vi "Doppler gating.vi"() -> ()   [LabVIEW 2022 SP3]
doc: "I. Description:\nThis example demonstrates how to use the timed loop to efficiently acquire a continuous amount of data (Waveform) using the DAQ devices internal clock and a counter to execute the timed loop only when all the data is available to Read.\n\nII. Instructions for Running:\n1. Select the physical channel to correspond to where your signal is input on the DAQ device. \n2. Enter the Source of Events. In this case we want the loop to execute on each AI sample clock pulse.\n3. Enter the counter you want to use to measure the events. In this example ctr0 is used as the default.\n4. Enter the minimum and maximum voltages.\nNote: For better accuracy try to match the input range to the expected voltage level of the measured signal.\n5. Select the number of samples to Read. Note: Because of the way this example uses the timed loop this parameter cannot be changed on-the-fly. \n6. Set the rate of the acquisition\nNote: The rate should be AT LEAST twice as fast as the maximum frequency component of the signal being acquired.\n\nIII. Block Diagram Steps:\n1. Create an Analog Input voltage channel.\n2. Set the timing type of the analog input task to Sample Clock. \n3. Call the DAQmx Create Timing Source (Digital Edge Counter) VI and specify the edge count to be the Samples to Read. What this does is cause the timed loop to only fire once it has received \"samples to read\" number of edges from the AI sample clock. This is an efficient use of CPU resources because the loop, and therefore the AI Read, will only execute once all of the samples are available.\n4. Call the Start VI to start the acquisition.\n5. Read the waveform once all the samples to read are available. In this approach the Read VI behaves in a \"non-blocking\" fashion, since it does not have to wait for samples to become available.\n6. Call the Clear Task VI to Clear the Task.\n7. Use the popup dialog box to display an error if any.\n\nIV. I/O Connections Overview:\nMake sure your signal input terminal matches the Physical Channel I/O Control. For further connection information, refer to your hardware reference manual."
uses:
  <vilib>/Utility/error.llb/DialogType.ctl
  <vilib>/Platform/TimedLoop/XDataNode/timing_clust.ctl
  <vilib>/Platform/TimedLoop/XDataNode/nitl_modes.ctl
  <vilib>/Platform/TimedLoop/XDataNode/wakeup.ctl
  <vilib>/DAQmx/read.llb/DAQmx Read.vi
  <vilib>/DAQmx/create/channels.llb/DAQmx Create Virtual Channel.vi
  <vilib>/DAQmx/configure/timing.llb/DAQmx Timing.vi
  <vilib>/DAQmx/create/timing.llb/DAQmx Create Timing Source.vi
  <vilib>/DAQmx/miscellaneous.llb/DAQmx Fill In Error Info.vi
  Instance          16 22Saved   Doppler gating .vi
  <vilib>/Platform/TimedLoop/XDataNode/XDataNode.xnode
  <vilib>/ptbypt/NI_PtbyPt.lvlib
  <vilib>/gmath/NI_Gmath.lvlib
  <vilib>/Platform/TimedLoop/XDataNode/XDNodeRunTimeDep.lvlib
panel:
  in  "window length":i32=500 caption="Samples to Read"
  in  "time increment":i32=100 caption="Samples to Read"
  out "Moving STFT":dbl[][](graph)
  in  "Counter":tag="Dev1/ctr0"
  in  "Source of Events":tag="/Dev1/ai/SampleClock"
  in  "Samples to Read":i32=1000
  in  "Physical Channel":tag="Dev1/ai0"
  in  "Minimum Value":dbl=-10.0 format="%0.2f"
  in  "Maximum Value":dbl=10.0 format="%0.2f"
  in  "stop":bool
  in  "Sample Rate":dbl=200000.0 caption="Sample Rate (Hz)" format="%0.2f"
  out "Measurement":waveform(dbl)[](graph)
  # "For instructions, select Help>>Show Context Help"
  # "Channel Parameters"
  # "Timing Parameters"
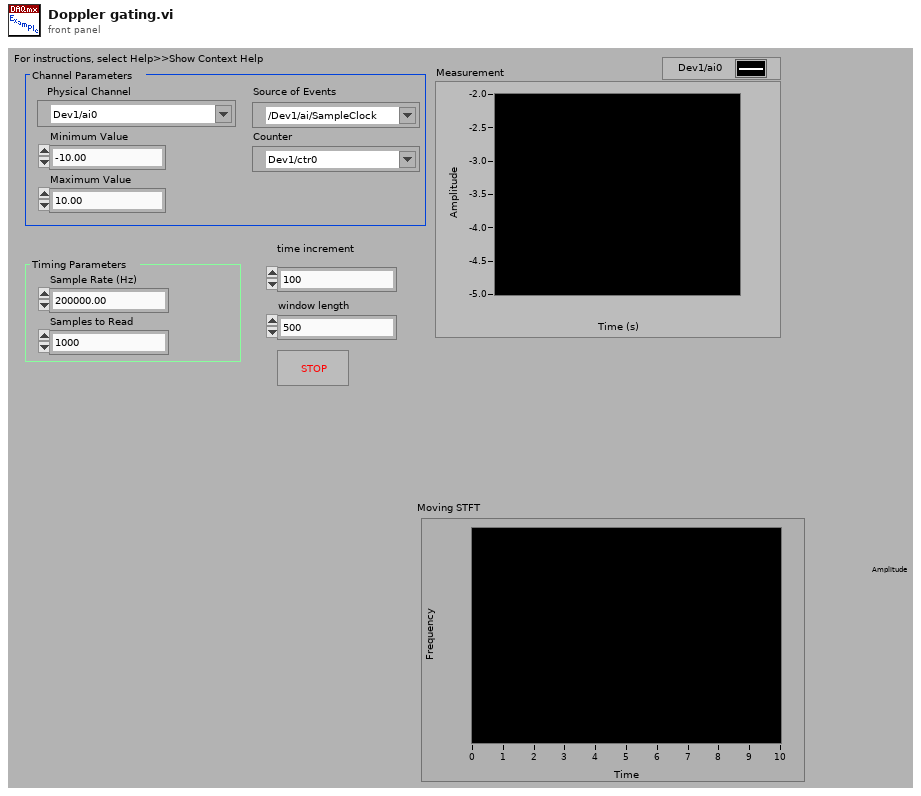
[diagram p1: front panel]
types:
  T1 = typedef "DialogType.ctl" = u16
  T2 = typedef "XDNodeRunTimeDep.lvlib/timing_clust.ctl" = cluster{"Expected End [f-1]":u64, "Actual End [f-1]":u64, "Finished Late? [f-1]":bool, "Expected End [i-1]":u64, "Actual End [i-1]":u64, "Finished Late? [i-1]":bool, "Expected Start [i]":u64, "Actual Start [i]":u64, "Expected Start [f]":u64, "Actual Start [f]":u64, "Source Name":string, "Structure Name":string, "Period":i64, "Deadline":i64, "Offset":i64, "Start":i64, "Priority":i32, "Timeout":i32, "Mode":T3, "Wakeup Reason":T4, "Error":errorcluster, "Source Type":string, "Secondary Source Type":string, "Global End Time":u64, "Global Start Time":u64, "Frame Duration":u64, "Iteration Duration":u64, "Assigned CPU":i32, "I/O Scan Engine Mode":u32}
  T3 = typedef "XDNodeRunTimeDep.lvlib/nitl_modes.ctl" = enum32{"No Change", "Process missed periods, maintain original phase", "Discard missed periods, maintain original phase", "Process missed periods, ignore original phase", "Discard missed periods, ignore original phase"}
  T4 = typedef "XDNodeRunTimeDep.lvlib/wakeup.ctl" = enum32{"Normal", "Aborted", "Asynchronous wakeup", "Timing source error", "Timed loop error", "Timeout"}
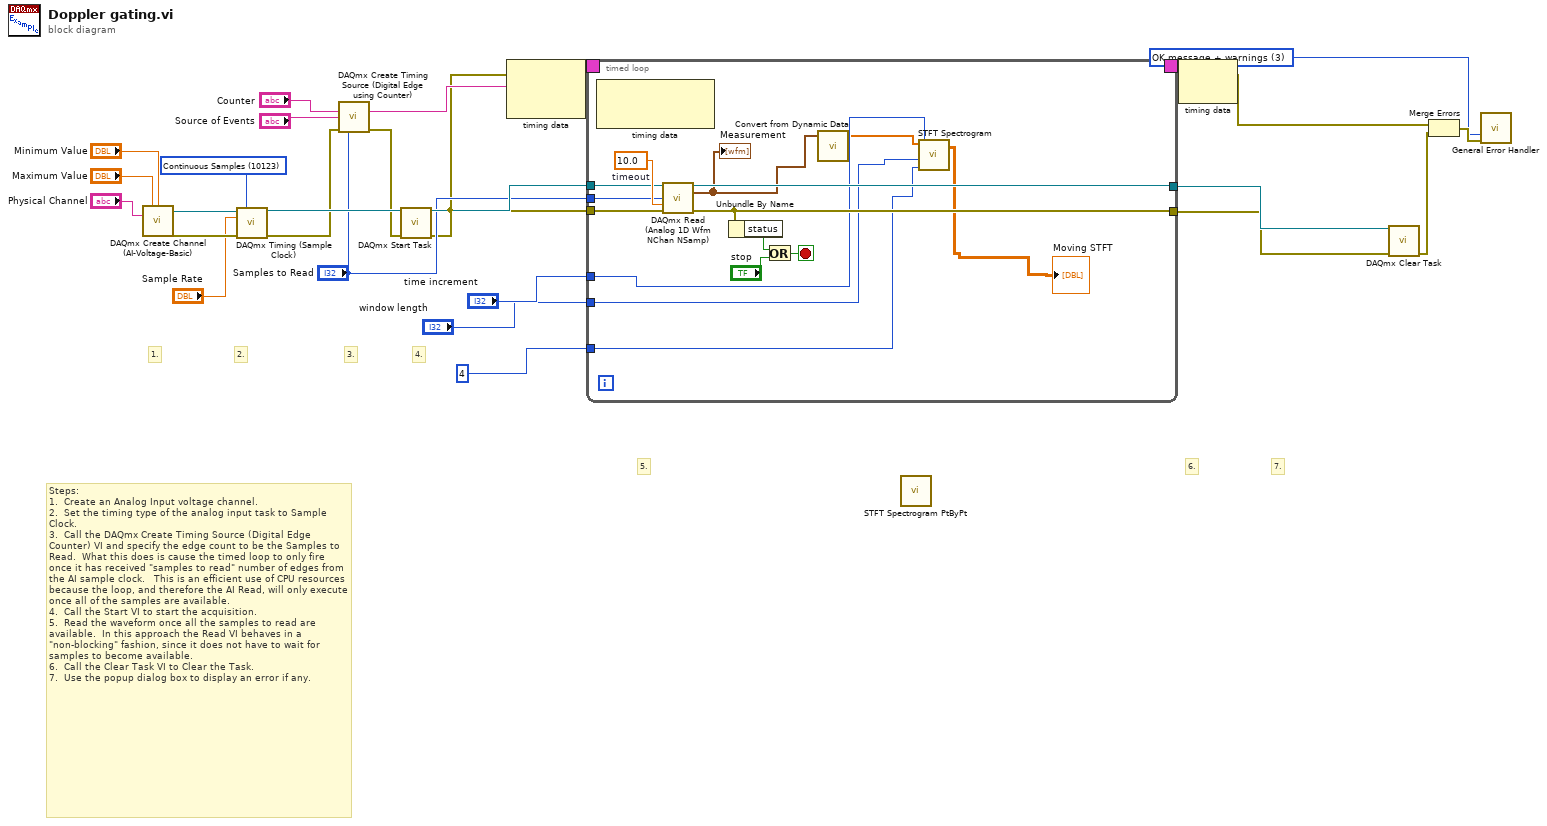
[diagram p0: block diagram]
diagram:
  w6 = T1 3 items=["no dialog", "OK message", "continue or stop message", "OK message + warnings", "continue/stop + warnings"] ("type of dialog (OK msg:1)")
  w21 = 10123 items=["Finite Samples"=10178, "Continuous Samples"=10123] ("sample mode")
  # "7."
  # "6."
  # "5."
  # "4."
  # "3."
  # "Steps:\n1.  Create an Analog Input voltage channel.\n2.  Set the timing type of the analog input task to Sample Clock. \n3.  Call the DAQmx Create Timing Source (Digital Edge Counter) VI and specify the edge count to be the Samples to Read.  What this does is cause the timed loop to only fire once it has received \"samples to read\" number of edges from the AI sample clock.   This is an efficient use of CPU resources because the loop, and therefore the AI Read, will only execute once all of the samples are available.\n4.  Call the Start VI to start the acquisition.\n5.  Read the waveform once all the samples to read are available.  In this approach the Read VI behaves in a \"non-blocking\" fashion, since it does not have to wait for samples to become available.\n6.  Call the Clear Task VI to Clear the Task.\n7.  Use the popup dialog box to display an error if any."
  # "1."
  # "2."
  n1 = call-poly <vilib>:"DAQmx Create Channel (AI-Voltage-Basic).vi"("maximum value"="Maximum Value", "minimum value"="Minimum Value", "physical channels"="Physical Channel") -> ("task out"=w24:refnum<k21>, "error out"=w25:errorcluster)  [unwired: 6 in, 5 out]
  n2 = call-poly <vilib>:"DAQmx Timing (Sample Clock).vi"("task/channels in"=w24, "sample mode"=w21, "rate"="Sample Rate", "error in"=w25) -> ("task out"=w18:refnum<k21>, "error out"=w17:errorcluster)  [unwired: 3 in, 7 out]
  n3 = call-poly <vilib>:"DAQmx Create Timing Source (Digital Edge using Counter).vi"("counter"="Counter", "source"="Source of Events", "error in"=w17, "edge count"="Samples to Read") -> ("timing source out"=w15:string, "error out"=w12:errorcluster)  [unwired: 3 in, 7 out]
  n4 = call <vilib>:"DAQmx Start Task.vi"("task/channels in"=w18, "error in"=w12) -> ("task out"=w16:refnum<k21>, "error out"=w10:errorcluster)  [unwired: 12 out]
  n5 = node-c288(w10, w15) -> (w1:T2)
  n6 = timed-loop {
    tunnel: 4 -> [w29]
    tunnel: "window length" -> [w30]
    tunnel: "time increment" -> [w31]
    tunnel: "Samples to Read" -> [w34]
    tunnel: w16 -> [w35]
    tunnel: w10 -> [w36]
    timing-out: [_] -> w2
    timing: w1 -> [_]
    tunnel: [w41] -> w20
    tunnel: [w42] -> w23
    stop <- w39 stop-if-true
    w37 = 10.0  # timeout
    n7 = node-c288() -> ()  [unwired: 3 out]
    n8 = call-poly <vilib>:"DAQmx Read (Analog 1D Wfm NChan NSamp).vi"("task/channels in"=w35, "number of samples per channel"=w34, "timeout"=w37, "error in"=w36) -> ("task out"=w42:refnum<k21>, "data"=w33:waveform(dbl)[], "error out"=w41:errorcluster)  [unwired: 9 out]
    "Measurement" <- w33
    n9 = Unbundle By Name(w41) -> ("status"=w40:bool)
    n10 = Or(x=w40, y="stop") -> (x .or. y?=w39:bool)
    n11 = call "Convert from Dynamic Data"("Dynamic Data Type"=w33) -> ("Array"=w28:dbl[])  [unwired: 3 out]
    n12 = call <vilib>:"STFT Spectrogram.vi"("window selector"=w29, "window length"=w30, "time increment"=w31, "X"=w28) -> ("STFT Spectrogram {X}"=→"Moving STFT":dbl[][])  [unwired: 1 out]
  }
  n13 = call <vilib>:"STFT Spectrogram PtByPt.vi"() -> ()  [unwired: 6 in, 2 out]
  n14 = node-c288(w2) -> (w9:errorcluster)
  n15 = call <vilib>:"DAQmx Clear Task.vi"("task in"=w23, "error in"=w20) -> ("error out"=w8:errorcluster)  [unwired: 13 out]
  n16 = Merge Errors(w9, w8) -> (w7:errorcluster)
  n17 = call <vilib>:"General Error Handler.vi"("type of dialog (OK msg:1)"=w6, "error in (no error)"=w7) -> ()  [unwired: 1 in, 13 out]
